vi "Auto settings.vi"(8 "error in (no error)":errorcluster, 10 "Array":dbl[](array[numeric]), 11 "Component Tray in":refnum<class "Component Tray.lvclass">) -> (0 "error out":errorcluster, 3 "Component Tray out":refnum<class "Component Tray.lvclass">)   [LabVIEW 2018, in "Component Tray.lvclass"]
uses:
  Component Tray.lvclass
  C:/Users/HEP/Documents/GitHub/New folder/C/Users/HEP/Documents/GitHub/UCSB-Gantry-HEP-2018/Classes/Workspace/Fixture.lvclass
  Fixture.lvclass/Fixture.ctl
  Write Gantry Region.vi
  Write Fixture ID.vi
  Write Position.vi
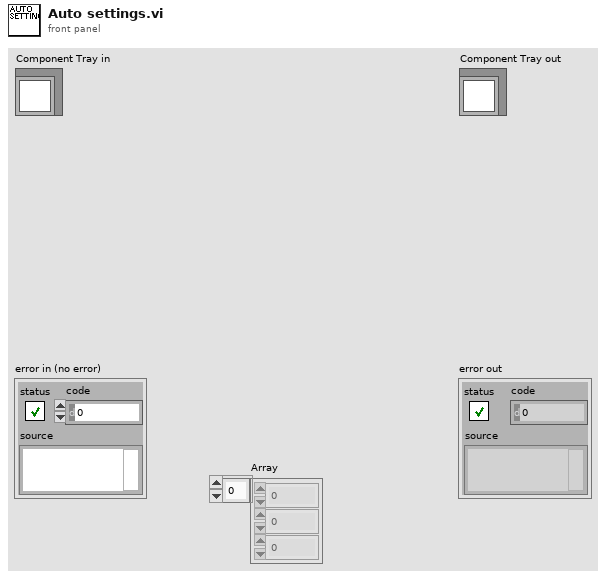
[diagram p1: front panel]
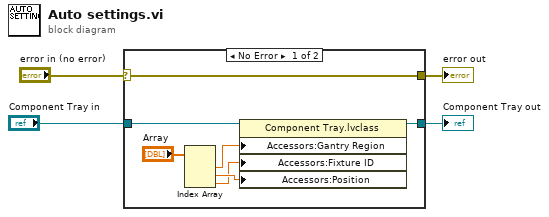
[diagram p0: block diagram]
diagram:
  n1 = case shown="No Error" "error in (no error)" {
    selector: "error in (no error)" -> [w11 w13]
    tunnel: [w11 w13] -> w3
    tunnel: [w9 w12] -> w1
    tunnel: "Component Tray in" -> [w10 w12]
    frame No Error {
      n2 = Index Array(array="Array") -> (element #1=w7:dbl, element #2=w6:dbl, element #3=w5:dbl)  [unwired: 3 in]
      n3 = property class="Component Tray.lvclass"(reference=w10, "Accessors:Gantry Region"=w7, "Accessors:Fixture ID"=w5, "Accessors:Position"=w6) -> (reference out=w9:refnum<class "Component Tray.lvclass">)  [unwired: 1 in, 1 out]
    }
    frame Error {
    }
  }
  "error out" <- w3
  "Component Tray out" <- w1
